vi "Create_blank_svg.vi"(0 "SVG Path":string="G:\\My Drive\\Nanosurf_data_processing\\Nanosurf_data\\2.25.2018\\InkscapeFiles\\2.25.2018.000000.svg", 5 "BMP for inkscape path":string="G:\\My Drive\\Nanosurf_data_processing\\Nanosurf_data\\2.25.2018\\bmpforinkscape\\2.25.2018.000000.bmp", 7 "HEIGHT":dbl=10.0 format="%#_13g", 9 "WIDTH":dbl format="%#_13g", 11 "error in":errorcluster) -> (4 "SVG Path Out":path, 15 "error out":errorcluster)   [LabVIEW 2020]
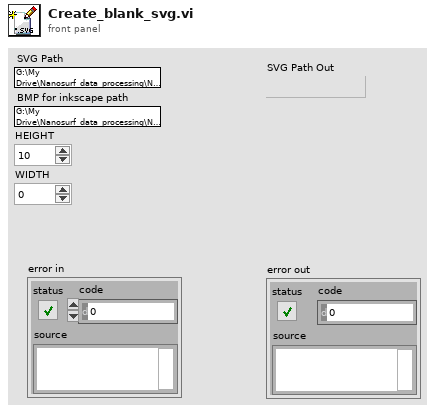
[diagram p1: front panel]
types:
  T1 = enum16{"open", "replace", "create", "open or create", "replace or create", "replace or create with confirmation"}
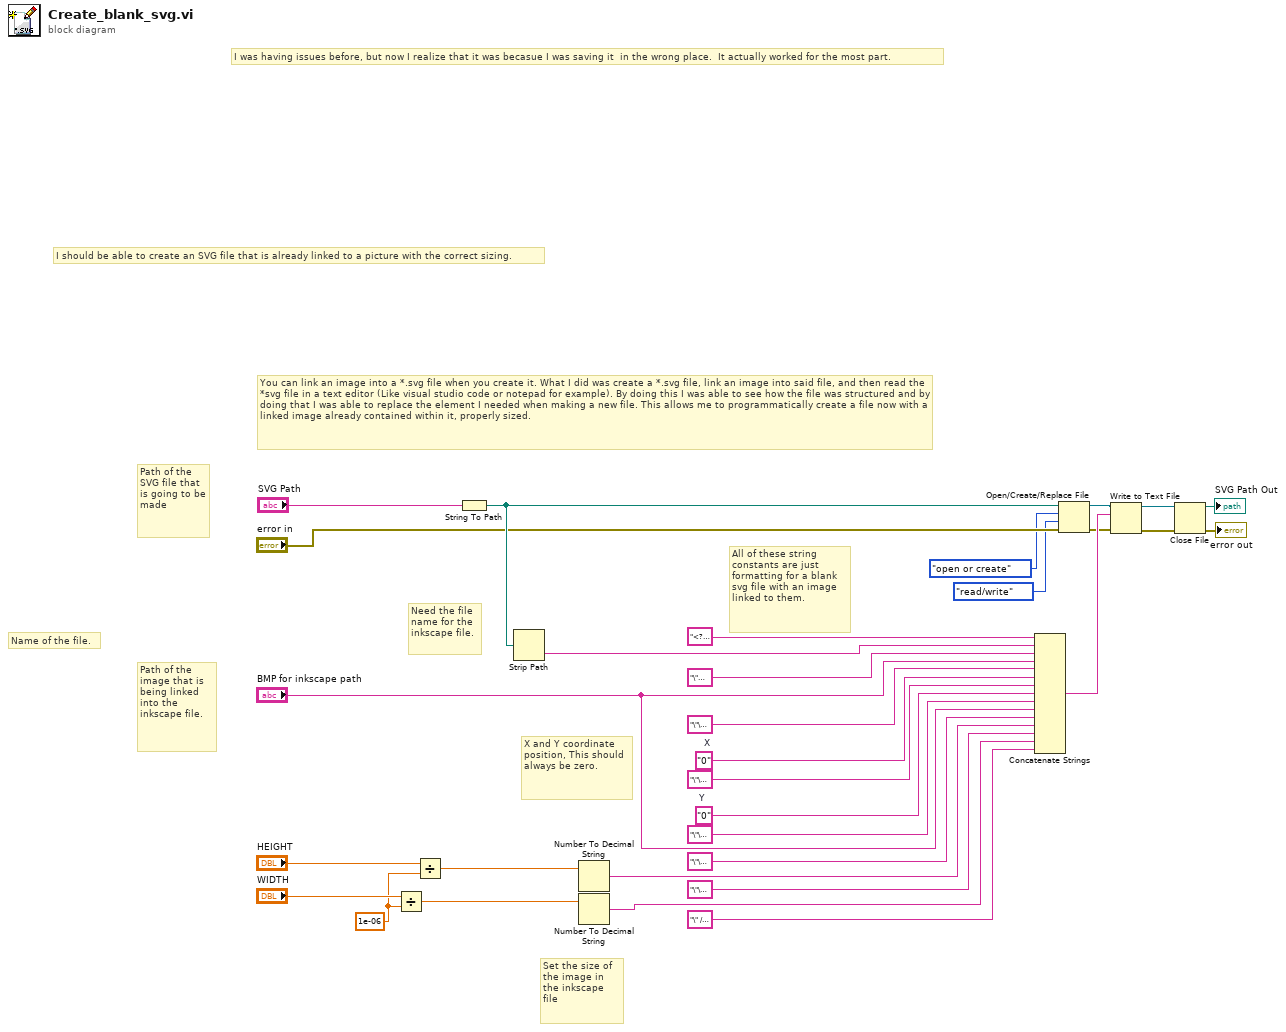
[diagram p0: block diagram]
diagram:
  w3 = 1e-06 ("y")
  w21 = "0"  # X
  w19 = "0"  # Y
  # "Need the file name for the inkscape file."
  # "All of these string constants are just formatting for a blank svg file with an image linked to them."
  # "Path of the SVG file that is going to be made"
  # "Path of the image that is being linked into the inkscape file."
  # "X and Y coordinate position, This should always be zero."
  # "Set the size of the image in the inkscape file"
  # "You can link an image into a *.svg file when you create it. What I did was create a *.svg file, link an image into said file, and then read the *svg file in a text editor (Like visual studio code or notepad for example). By doing this I was able to see how the file was structured and by doing that I was able to replace the element I needed when making a new file. This allows me to programmatically create a file now with a linked image already contained within it, properly sized."
  # "I was having issues before, but now I realize that it was becasue I was saving it  in the wrong place.  It actually worked for the most part."
  # "I should be able to create an SVG file that is already linked to a picture with the correct sizing."
  # "Name of the file."
  n1 = Divide(x="WIDTH", y=w3) -> (x/y=w4:dbl)
  n2 = Divide(x="HEIGHT", y=w3) -> (x/y=w1:dbl)
  n3 = String To Path(string="SVG Path") -> (path=w29:path)
  n4 = Strip Path(path=w29) -> (name=w12:string)  [unwired: 1 out]
  n5 = Number To Decimal String(number=w1) -> (decimal integer string=w17:string)  [unwired: 1 in]
  n6 = Number To Decimal String(number=w4) -> (decimal integer string=w11:string)  [unwired: 1 in]
  n7 = Concatenate Strings("<?xml version=\"1.0\" encoding=\"UTF-8\" standalone=\"no\"?>\n<!-- Created with Inkscape (http://www.inkscape.org/) -->\n\n<svg\n   xmlns:dc=\"http://purl.org/dc/elements/1.1/\"\n   xmlns:cc=\"http://creativecommons.org/ns#\"\n   xmlns:rdf=\"http://www.w3.org/1999/02/22-rdf-syntax-ns#\"\n   xmlns:svg=\"http://www.w3.org/2000/svg\"\n   xmlns=\"http://www.w3.org/2000/svg\"\n   xmlns:xlink=\"http://www.w3.org/1999/xlink\"\n   xmlns:sodipodi=\"http://sodipodi.sourceforge.net/DTD/sodipodi-0.dtd\"\n   xmlns:inkscape=\"http://www.inkscape.org/namespaces/inkscape\"\n   width=\"210mm\"\n   height=\"297mm\"\n   viewBox=\"0 0 210 297\"\n   version=\"1.1\"\n   id=\"svg8\"\n   inkscape:version=\"0.92.2 (5c3e80d, 2017-08-06)\"\n   sodipodi:docname=\"", w12, "\">\n  <defs\n     id=\"defs2\" />\n  <sodipodi:namedview\n     id=\"base\"\n     pagecolor=\"#ffffff\"\n     bordercolor=\"#666666\"\n     borderopacity=\"1.0\"\n     inkscape:pageopacity=\"0.0\"\n     inkscape:pageshadow=\"2\"\n     inkscape:zoom=\"0.0875\"\n     inkscape:cx=\"-3419.1375\"\n     inkscape:cy=\"-153.35601\"\n     inkscape:document-units=\"mm\"\n     inkscape:current-layer=\"layer1\"\n     showgrid=\"false\"\n     inkscape:window-width=\"1600\"\n     inkscape:window-height=\"837\"\n     inkscape:window-x=\"-8\"\n     inkscape:window-y=\"-8\"\n     inkscape:window-maximized=\"1\" />\n  <metadata\n     id=\"metadata5\">\n    <rdf:RDF>\n      <cc:Work\n         rdf:about=\"\">\n        <dc:format>image/svg+xml</dc:format>\n        <dc:type\n           rdf:resource=\"http://purl.org/dc/dcmitype/StillImage\" />\n        <dc:title />\n      </cc:Work>\n    </rdf:RDF>\n  </metadata>\n  <g\n     inkscape:label=\"Layer 1\"\n     inkscape:groupmode=\"layer\"\n     id=\"layer1\">\n    <image\n       sodipodi:absref=\"", "BMP for inkscape path", "\"\n       y=\"", w21, "\"\n       x=\"", w19, "\"\n       id=\"image16\"\n       xlink:href=\"file:///", "BMP for inkscape path", "\"\n       preserveAspectRatio=\"none\"\n       height=\"", w17, "\"\n       width=\"", w11, "\" />\n  </g>\n</svg>") -> (w27:string)
  n8 = Open/Create/Replace File(file path (use dialog)=w29, error in="error in", operation (0:open)=T1."open or create", access (0:read/write)=enum16{"read/write", "read-only", "write-only"}."read/write") -> (refnum out=w28:refnum<file>, error out=w26:errorcluster)  [unwired: 2 in, 1 out]
  n9 = Write to Text File(file (use dialog)=w28, text=w27, error in=w26) -> (refnum out=w25:refnum<file>, error out=w24:errorcluster)  [unwired: 1 in, 1 out]
  n10 = Close File(refnum=w25, error in=w24) -> (path=→"SVG Path Out":path, error out=→"error out":errorcluster)
